vi "Launch.vi"(8 "error in (no error)":errorcluster, 11 "Flex UI (Actor) in":refnum<class "Flex UI (Actor).lvclass">) -> (0 "error out":errorcluster, 3 "Flex UI (Actor) out":refnum<class "Flex UI (Actor).lvclass">)   [LabVIEW 2016, in "Flex UI (Parent Actor).lvlib" / "Flex UI (Actor).lvclass"]
doc: "Wrapper around the Launch method from the Flex UI class."
uses:
  Flex UI (Actor).lvclass
  <vilib>/East West Architects/Flex UI/Flex UI (Parent)/Flex UI.lvclass
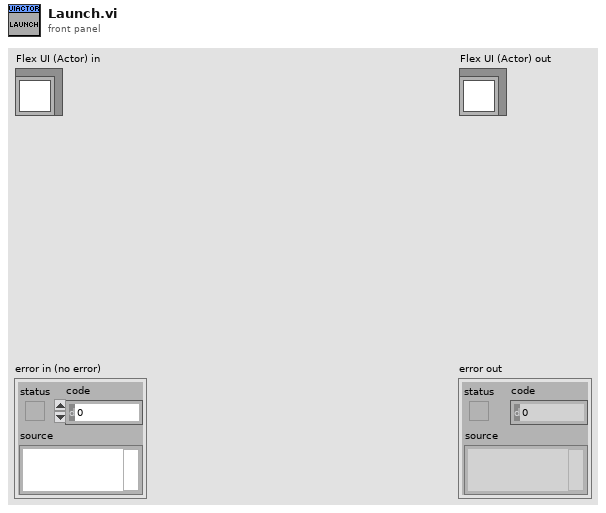
[diagram p1: front panel]
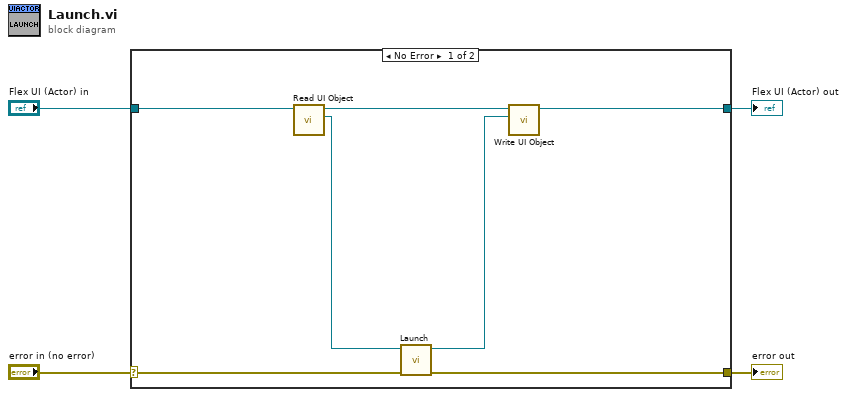
[diagram p0: block diagram]
diagram:
  n1 = case shown="No Error" "error in (no error)" {
    selector: "error in (no error)" -> [w10 w13]
    tunnel: [w9 w13] -> w3
    tunnel: [w7 w12] -> w1
    tunnel: "Flex UI (Actor) in" -> [w11 w12]
    frame No Error {
      n2 = call-dynamic "Read UI Object.vi"("Flex UI (Actor) in"=w11) -> ("Flex UI Object"=w6:refnum<class "Flex UI.lvclass">, "Flex UI (Actor) out"=w8:refnum<class "Flex UI (Actor).lvclass">)  [unwired: 8 in, 1 out]
      n3 = call-dynamic "Launch.vi"("error in"=w10, "Flex UI in"=w6) -> ("error out"=w9:errorcluster, "Flex UI out"=w5:refnum<class "Flex UI.lvclass">)  [unwired: 8 in]
      n4 = call-dynamic "Write UI Object.vi"("Flex UI in"=w5, "Flex UI (Actor) in"=w8) -> ("Flex UI (Actor) out"=w7:refnum<class "Flex UI (Actor).lvclass">)  [unwired: 8 in, 1 out]
    }
    frame Error {
    }
  }
  "error out" <- w3
  "Flex UI (Actor) out" <- w1
